vi "ExpressVI.vi"(8 "Action":enum16{"Addition", "Multiplication"}(ring), 10 "B":dbl, 11 "A":dbl) -> (3 "Result":dbl)   [LabVIEW 2023]
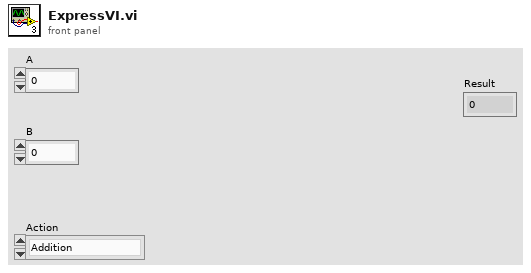
[diagram p1: front panel]
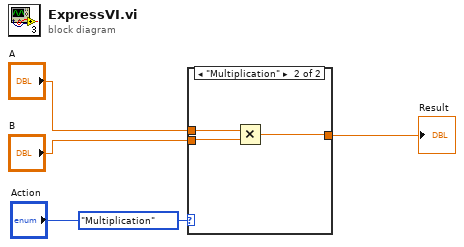
[diagram p0: block diagram]
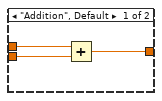
[diagram p2: hidden frame]
diagram:
  (unwired) enum16{"Addition", "Multiplication"}."Multiplication" ("Action")
  n1 = case shown="\"Multiplication\"" "Action" {
    tunnel: "A" -> [w7 w9]
    tunnel: "B" -> [w6 w8]
    tunnel: [w5 w10] -> w1
    frame "Addition", Default {
      n2 = Add(x=w7, y=w6) -> (x+y=w5:dbl)
    }
    frame "Multiplication" {
      n3 = Multiply(x=w9, y=w8) -> (x*y=w10:dbl)
    }
  }
  "Result" <- w1
